vi "LV_File_Start.vi"(8 "error in":errorcluster, 10 "VI Name":string, 11 "LV_File.lvclass (IN)":refnum<class "LV_File.lvclass">) -> (0 "error out":errorcluster, 3 "LV_File.lvclass (OUT)":refnum<class "LV_File.lvclass">)   [LabVIEW 2013, in "LV_File.lvclass"]
uses:
  LV_File.lvclass
  LV_File.lvclass/LV_File.ctl
  File.lvclass
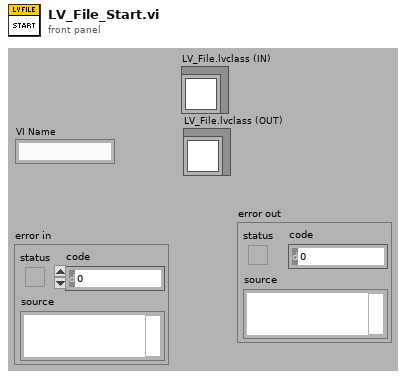
[diagram p1: front panel]
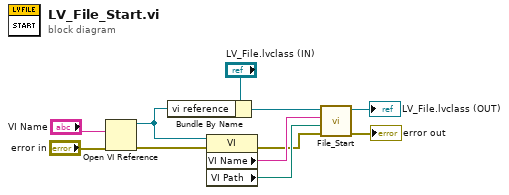
[diagram p0: block diagram]
diagram:
  n1 = Open VI Reference(vi path="VI Name", error in (no error)="error in") -> (vi reference=w3:refnum<vi>, error out=w8:errorcluster)  [unwired: 4 in]
  n2 = Bundle By Name(cluster="LV_File.lvclass (IN)", "vi reference"=w3) -> (w10:refnum<class "LV_File.lvclass">)
  n3 = property class="VI"(reference=w3, error in=w8) -> (error out=w2:errorcluster, "VI Name"=w6:string, "VI Path"=w5:path)  [unwired: 1 out]
  n4 = call "File_Start.vi"("error in"=w2, "Path"=w5, "Name"=w6, "File.lvclass (IN)"=w10) -> ("error out"=→"error out":errorcluster, "File.lvclass (OUT)"=→"LV_File.lvclass (OUT)":refnum<class "LV_File.lvclass">)  [unwired: 6 in]
